vi "Sensor to Certainty graph.vi"(6 "Distance":fxp<+/-,64,32>, 8 "Degrees":dbl, 9 "Sensor y":i16, 10 "Sensor x":i16, 11 "Array 2":i16[][](array[numeric])) -> (3 "Array 3":i16[][](array[numeric]))   [LabVIEW 2012]
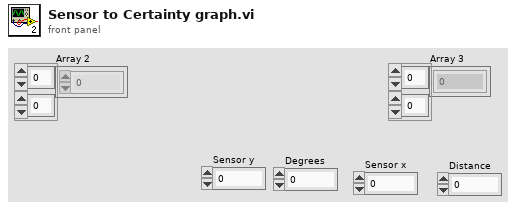
[diagram p1: front panel]
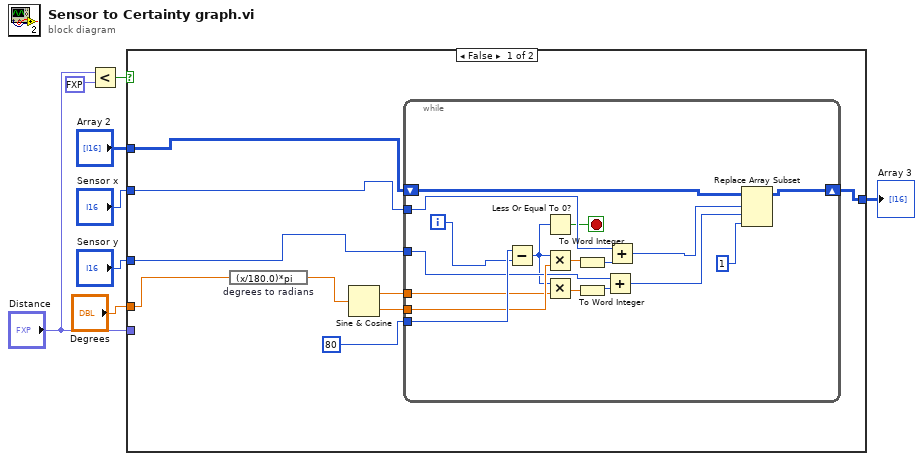
[diagram p0: block diagram]
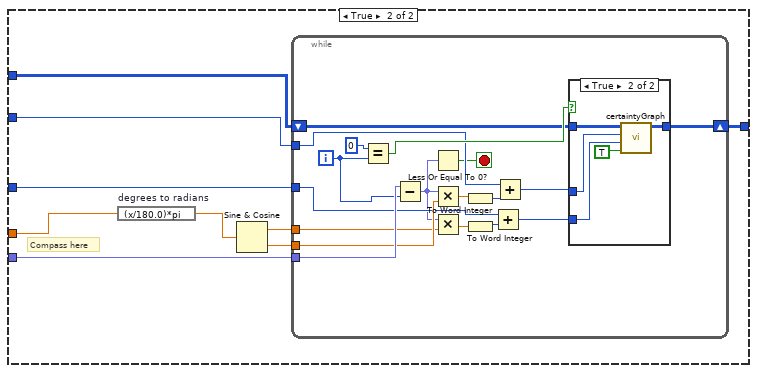
[diagram p2: hidden frame]
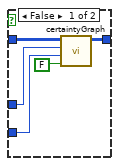
[diagram p3: hidden frame]
diagram:
  n1 = Less?(x="Distance", y=fxp<+/-,64,32> 80.0) -> (x < y?=w5:bool)
  n2 = case shown="False" w5 {
    tunnel: "Array 2" -> [w14 w40]
    tunnel: [w13 w39] -> w7
    tunnel: "Distance" -> [_ w38]
    tunnel: "Sensor x" -> [w11 w37]
    tunnel: "Sensor y" -> [w10 w36]
    tunnel: "Degrees" -> [w9 w35]
    frame False {
      n3 = expression code="(x/180.0)*pi" "degrees to radians"(w9) -> (w17:dbl)
      n4 = Sine & Cosine(0:w17) -> (1:w16:dbl, 2:w15:dbl)
      n5 = while {
        tunnel: w10 -> [w31]
        tunnel: w11 -> [w30]
        tunnel: 80 -> [w34]
        tunnel: w16 -> [w32]
        tunnel: w15 -> [w33]
        shift-right: [w22] -> w13
        shift-left: w14 -> [w23]
        i -> [w18]
        stop <- w28 stop-if-true
        n6 = Subtract(x=w34, y=w18) -> (x-y=w29:i32)
        n7 = Less Or Equal To 0?(x=w29) -> (x <= 0?=w28:bool)
        n8 = Multiply(x=w29, y=w33) -> (x*y=w27:dbl)
        n9 = Multiply(x=w29, y=w32) -> (x*y=w24:dbl)
        n10 = To Word Integer(number=w27) -> (16bit integer=w26:i16)
        n11 = To Word Integer(number=w24) -> (16bit integer=w25:i16)
        n12 = Add(x=w31, y=w25) -> (x+y=w20:i16)
        n13 = Add(x=w30, y=w26) -> (x+y=w21:i16)
        n14 = Replace Array Subset(array=w23, new element=1, index (row)=w21, index (col)=w20) -> (w22:i16[][])
      }
    }
    frame True {
      # "Compass here"
      n15 = expression code="(x/180.0)*pi" "degrees to radians"(w35) -> (w43:dbl)
      n16 = Sine & Cosine(0:w43) -> (1:w42:dbl, 2:w41:dbl)
      n17 = while {
        tunnel: w36 -> [w56]
        tunnel: w37 -> [w55]
        tunnel: w38 -> [w59]
        tunnel: w42 -> [w57]
        tunnel: w41 -> [w58]
        shift-right: [w51] -> w39
        shift-left: w40 -> [w54]
        i -> [w44]
        stop <- w52 stop-if-true
        n18 = Equal?(x=0, y=w44) -> (x = y?=w60:bool)
        n19 = Subtract(x=w59, y=w44) -> (x-y=w53:fxp<+/-,64,33>)
        n20 = Less Or Equal To 0?(x=w53) -> (x <= 0?=w52:bool)
        n21 = Multiply(x=w53, y=w58) -> (x*y=w50:dbl)
        n22 = Multiply(x=w53, y=w57) -> (x*y=w45:dbl)
        n23 = To Word Integer(number=w50) -> (16bit integer=w49:i16)
        n24 = To Word Integer(number=w45) -> (16bit integer=w46:i16)
        n25 = Add(x=w56, y=w46) -> (x+y=w47:i16)
        n26 = Add(x=w55, y=w49) -> (x+y=w48:i16)
        n27 = case shown="True" w60 {
          tunnel: w48 -> [w66 w70]
          tunnel: w47 -> [w65 w69]
          tunnel: w54 -> [w63 w68]
          tunnel: [w62 w67] -> w51
          frame False {
            n28 = call "certaintyGraph.vi"("Detected"=FALSE, "Y"=w65, "X"=w66, "Array"=w63) -> ("Array 2"=w62:i16[][])  [unwired: 7 in]
          }
          frame True {
            n29 = call "certaintyGraph.vi"("Detected"=TRUE, "Y"=w69, "X"=w70, "Array"=w68) -> ("Array 2"=w67:i16[][])  [unwired: 7 in]
          }
        }
      }
    }
  }
  "Array 3" <- w7
